vi "IOUpdate.vi"(8 "error in (no error)":errorcluster, 11 "VISA Reference":refnum<visa-resource-name>) -> (0 "error out":errorcluster, 3 "dup VISA resource name":refnum<visa-resource-name>)   [LabVIEW 2016]
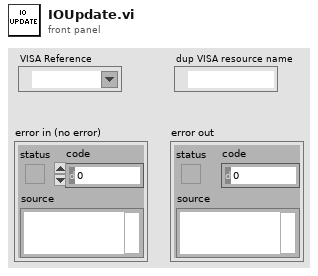
[diagram p1: front panel]
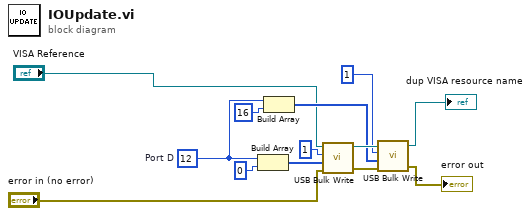
[diagram p0: block diagram]
diagram:
  w11 = u8 12  # Port D
  n1 = Build Array(w11, u8 0 ("x")) -> (w8:u8[])
  n2 = Build Array(w11, u8 16 ("x")) -> (w6:u8[])
  n3 = call "USB Bulk Write.vi"("error in (no error)"="error in (no error)", "message"=w8, "Endpoint"=i16 1, "VISA Reference"="VISA Reference") -> ("error out"=w13:errorcluster, "dup VISA resource name"=w12:refnum<visa-resource-name>)  [unwired: 1 out]
  n4 = call "USB Bulk Write.vi"("error in (no error)"=w13, "message"=w6, "Endpoint"=i16 1, "VISA Reference"=w12) -> ("error out"=→"error out":errorcluster, "dup VISA resource name"=→"dup VISA resource name":refnum<visa-resource-name>)  [unwired: 1 out]
